vi "Editor Soglie.vi"(6 "delimiter":string="::", 7 "Grandezze misurate":string[](array[string]), 8 "file path Soglie int":path=path "C:/Lavori in corso/C2014015_CDR_PumpTEST/PC/Codice/Settings/Tolleranze misure/SoglieQH int.txt", 9 "file path Soglie costanti":path=path "C:/Lavori in corso/C2014015_CDR_PumpTEST/PC/Codice/Settings/Tolleranze misure/Soglie QH.txt", 10 "file path Soglie AQ int":path=path "C:/Lavori in corso/C2014015_CDR_PumpTEST/PC/Codice/Settings/Tolleranze misure/Soglie AQ QH int.txt", 11 "file path Soglie AQ costanti":path=path "C:/Lavori in corso/C2014015_CDR_PumpTEST/PC/Codice/Settings/Tolleranze misure/Soglie AQ QH.txt") -> (0 "Array soglie interpolate":T1(array[cluster]), 1 "Array soglie costanti":T2(array[cluster])=[{"Grandezza"="", "colonna"=1, "upper limit"=50.5, "misura"=0.0, "lower limit"=49.5, "Allarme?"=FALSE, "Inizio"=timestamp(0 s since 1904-01-01), "Durata [s]"=0.0}, {"Grandezza"="", "colonna"=2, "upper limit"=240.0, "misura"=0.0, "lower limit"=220.0, "Allarme?"=FALSE, "Inizio"=timestamp(0 s since 1904-01-01), "Durata [s]"=0.0}, {"Grandezza"="", "colonna"=3, "upper limit"=3.0, "misura"=0.0, "lower limit"=0.0, "Allarme?"=FALSE, "Inizio"=timestamp(0 s since 1904-01-01), "Durata [s]"=0.0}], 2 "Soglie AQ interpolate":T3(array[cluster]), 3 "Soglie AQ costanti":T4(array[cluster]))   [LabVIEW 2016]
uses:
  <vilib>/Utility/file.llb/Read From Spreadsheet File (string).vi
  <vilib>/Utility/file.llb/Write To Spreadsheet File (string).vi
  <vilib>/Utility/file.llb/Write To Spreadsheet File (DBL).vi
panel:
  in  "Intervento\nsoglie":bool caption="Soglia costante\n\nSoglia interpolata"
  out "Grandezza\nselezionata":string
  in  "Selezione\nsoglie":bool caption="Soglia costante\n\nSoglia interpolata"
  in  "Stop":bool
  in  "Soglia":T5 caption="Soglia costante"
  in  "Soglia interpolata":T6 caption="Soglia dinamica"
  in  "Grandezze misurate":i32(listbox)
  # "Soglie costanti"
  # "Soglie dinamiche"
  # "Solo acquisizione"
  # "Sempre attivo"
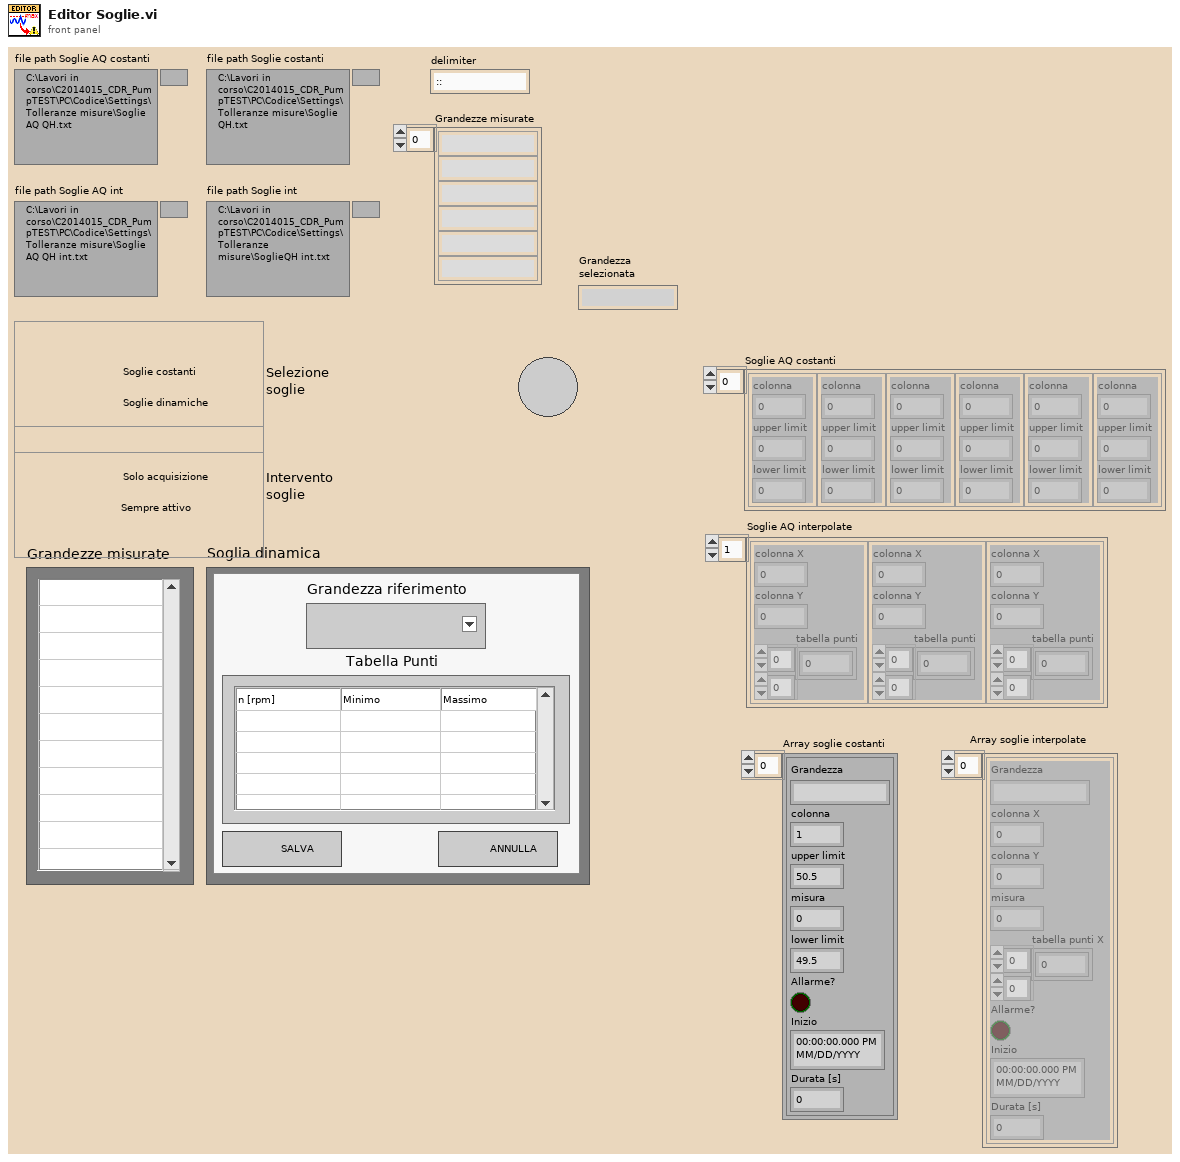
[diagram p1: front panel]
types:
  T1 = cluster{"Grandezza":string, "colonna X":i32, "colonna Y":i32, "misura":dbl, "tabella punti X":dbl[][], "Allarme?":bool, "Inizio":timestamp, "Durata [s]":dbl}[]
  T2 = cluster{"Grandezza":string, "colonna":i32, "upper limit":dbl, "misura":dbl, "lower limit":dbl, "Allarme?":bool, "Inizio":timestamp, "Durata [s]":dbl}[]
  T3 = cluster{"colonna X":i32, "colonna Y":i32, "tabella punti":dbl[][]}[]
  T4 = cluster{"colonna":i32, "upper limit":dbl, "lower limit":dbl}[]
  T5 = cluster{"Limite Massimo":dbl, "Limite Minimo":dbl, "Ok":bool, "ANNULLA":bool}
  T6 = cluster{"Tabella Punti":string[][], "Ok":bool, "ANNULLA":bool, "Grandezza riferimento":u16}
  T7 = cluster{"colonna X":i32, "colonna Y":i32, "tabella punti":dbl[][]}
  T8 = cluster{"colonna":i32, "upper limit":dbl, "lower limit":dbl}
  T9 = cluster{"Grandezza":string, "colonna X":i32, "colonna Y":i32, "misura":dbl, "tabella punti X":dbl[][], "Allarme?":bool, "Inizio":timestamp, "Durata [s]":dbl}
  T10 = cluster{"Grandezza":string, "colonna":i32, "upper limit":dbl, "misura":dbl, "lower limit":dbl, "Allarme?":bool, "Inizio":timestamp, "Durata [s]":dbl}
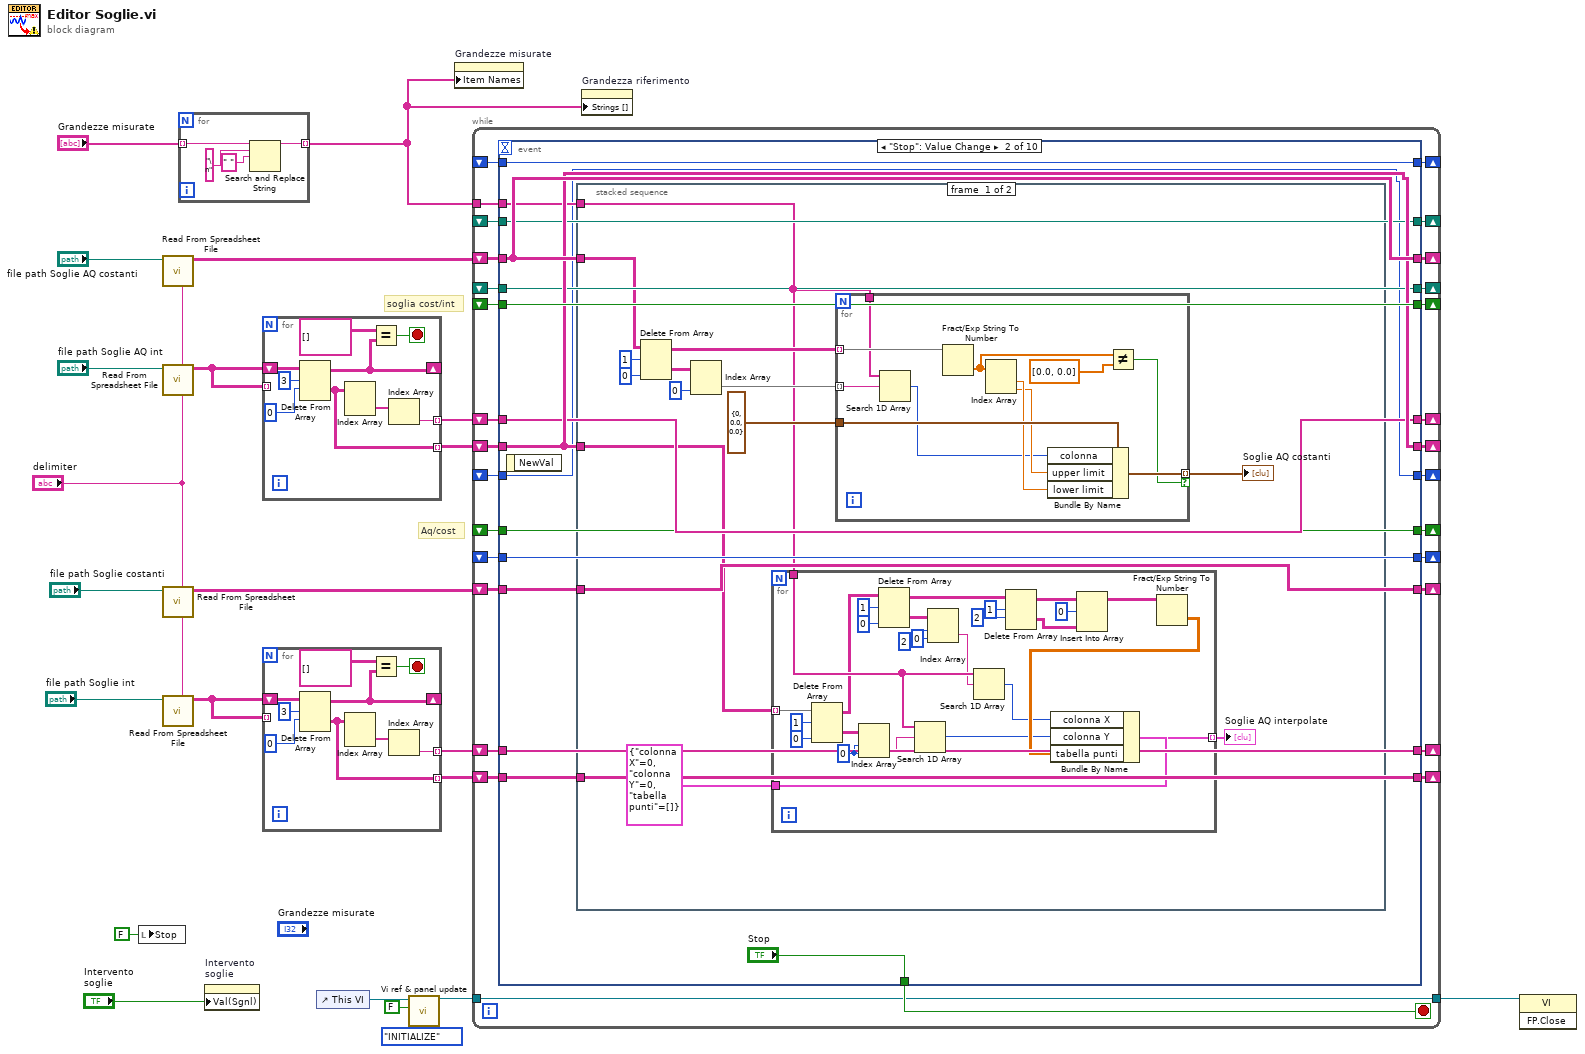
[diagram p0: block diagram]
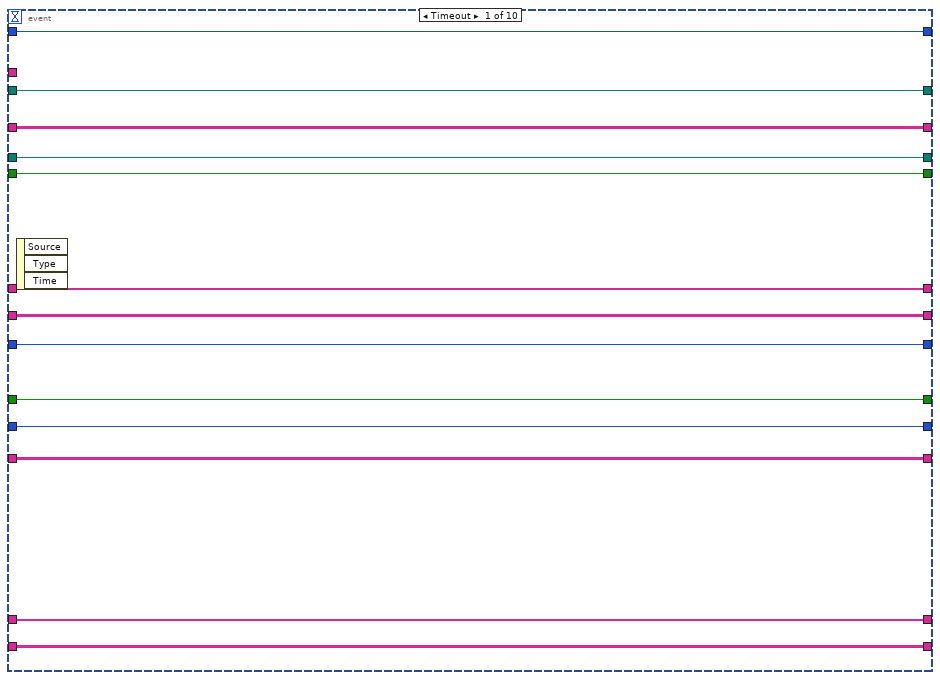
[diagram p2: hidden frame]
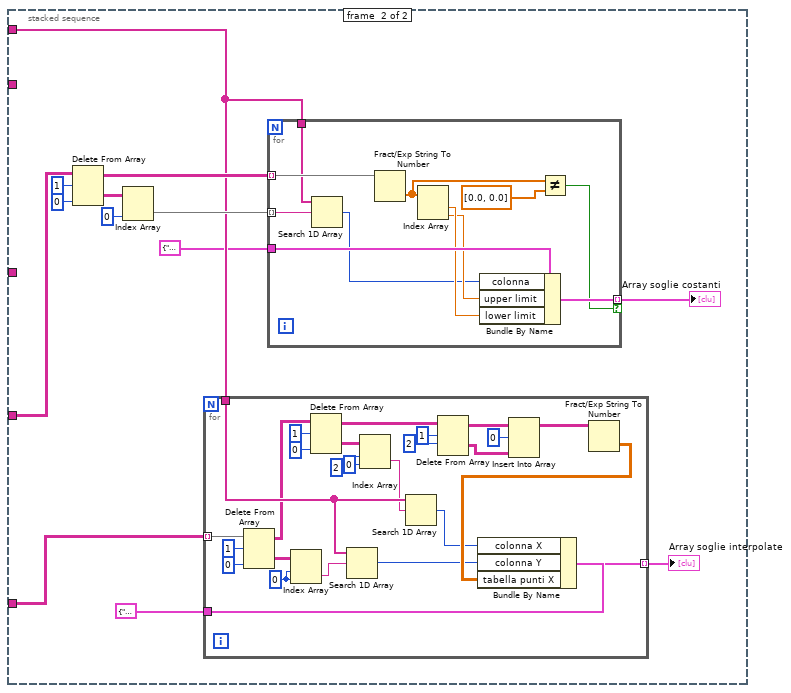
[diagram p3: hidden frame]
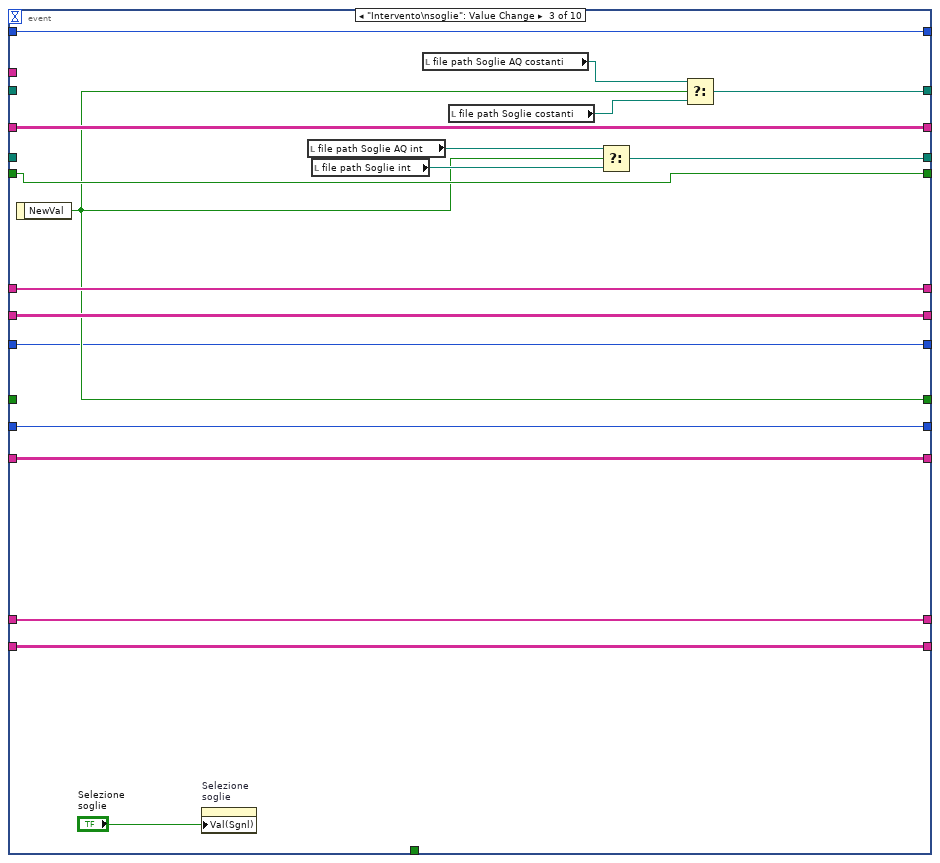
[diagram p4: hidden frame]
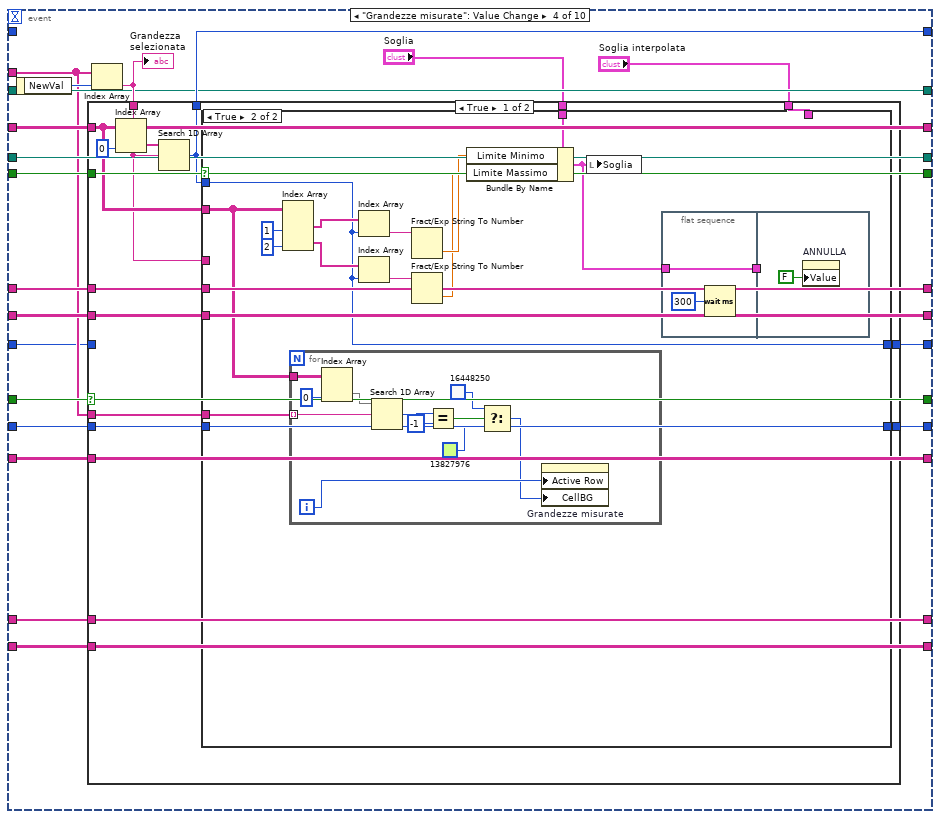
[diagram p5: hidden frame]
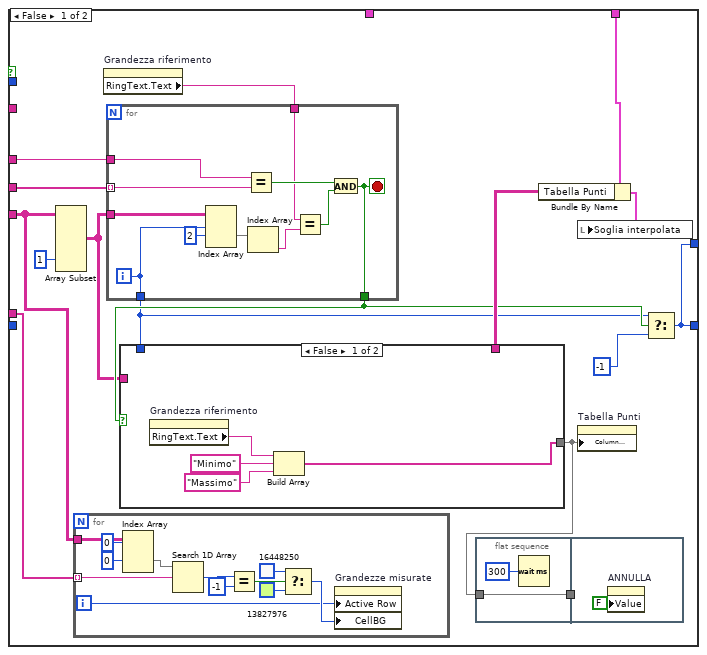
[diagram p6: hidden frame]
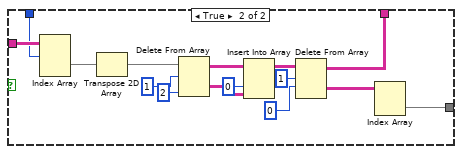
[diagram p7: hidden frame]
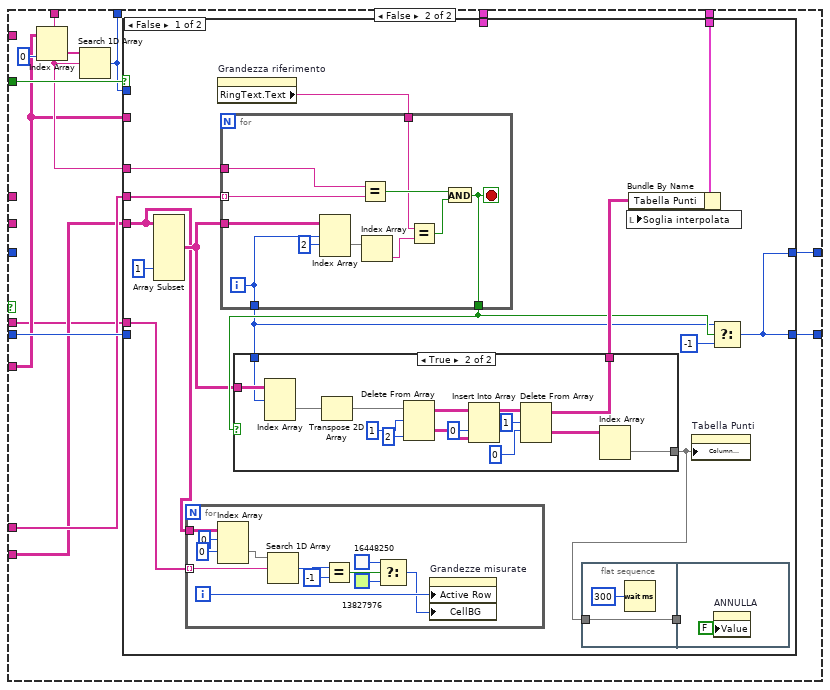
[diagram p8: hidden frame]
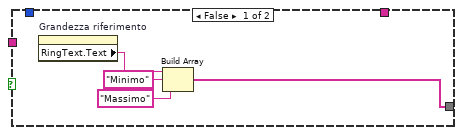
[diagram p9: hidden frame]
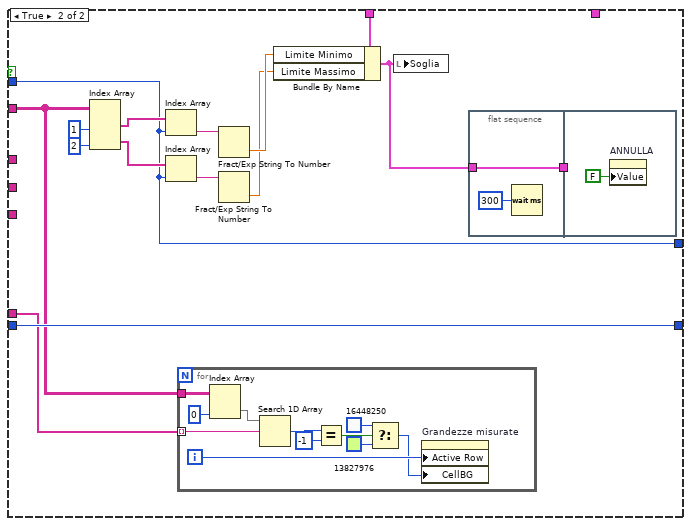
[diagram p10: hidden frame]
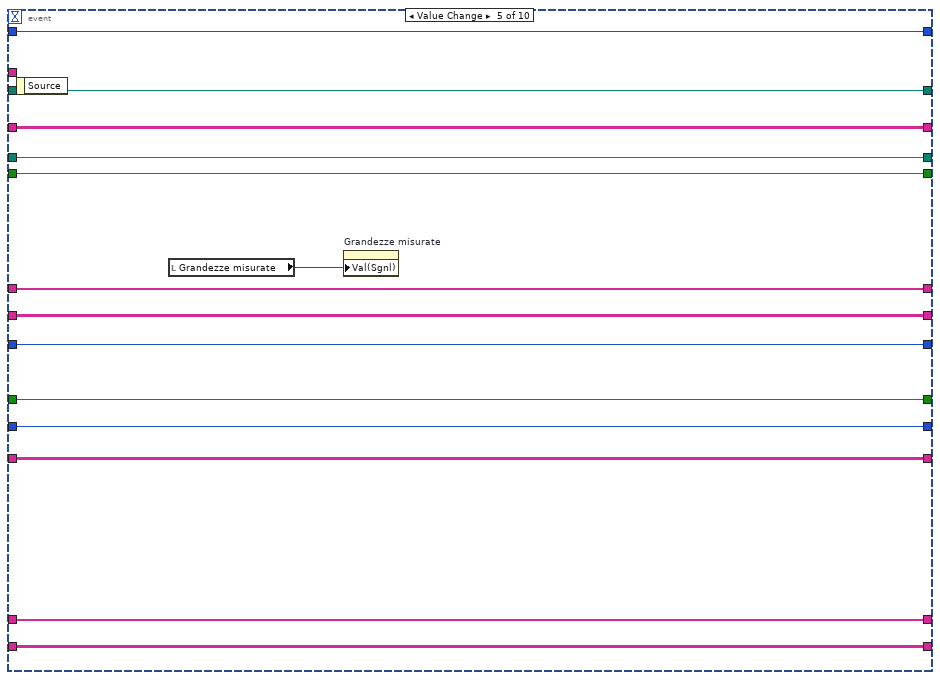
[diagram p11: hidden frame]
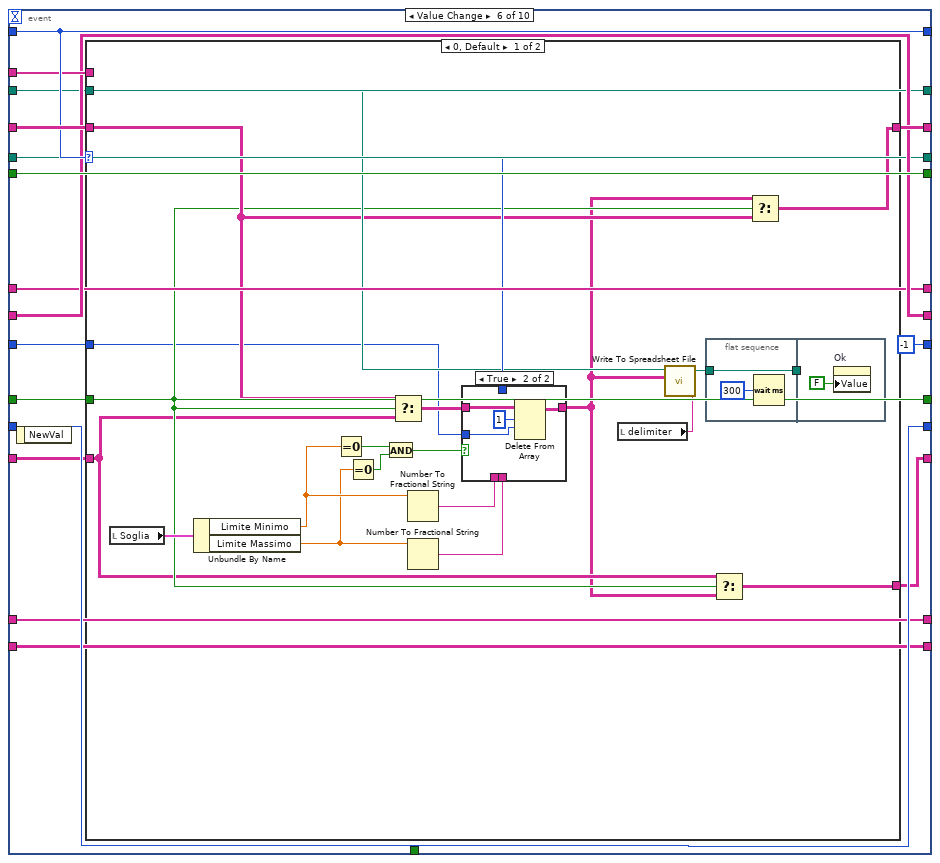
[diagram p12: hidden frame]
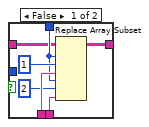
[diagram p13: hidden frame]
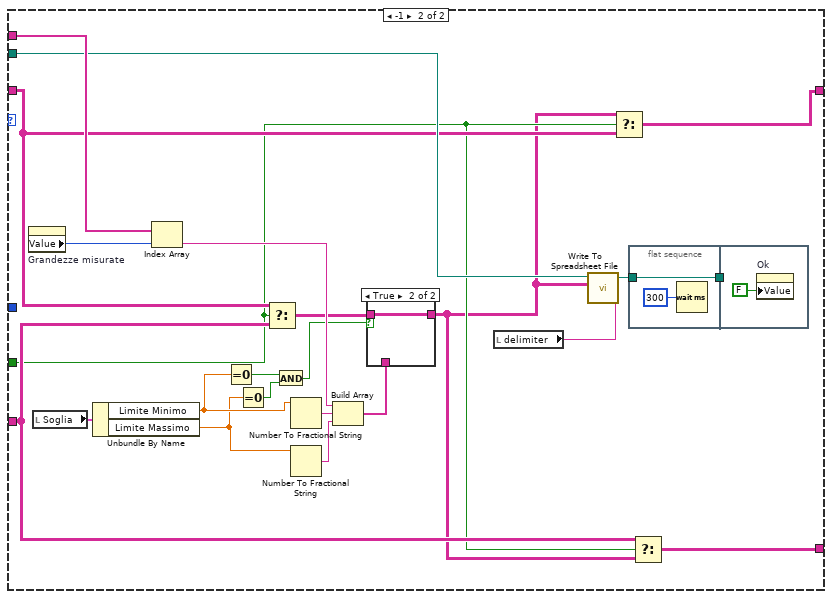
[diagram p14: hidden frame]
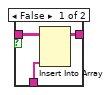
[diagram p15: hidden frame]
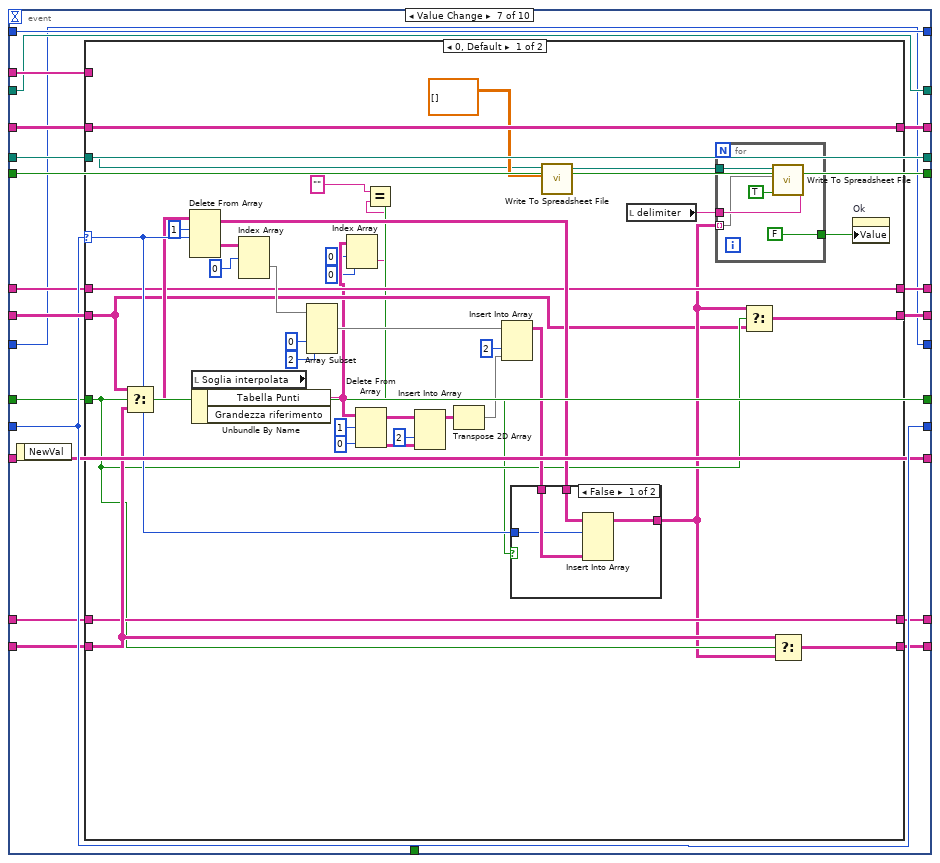
[diagram p16: hidden frame]
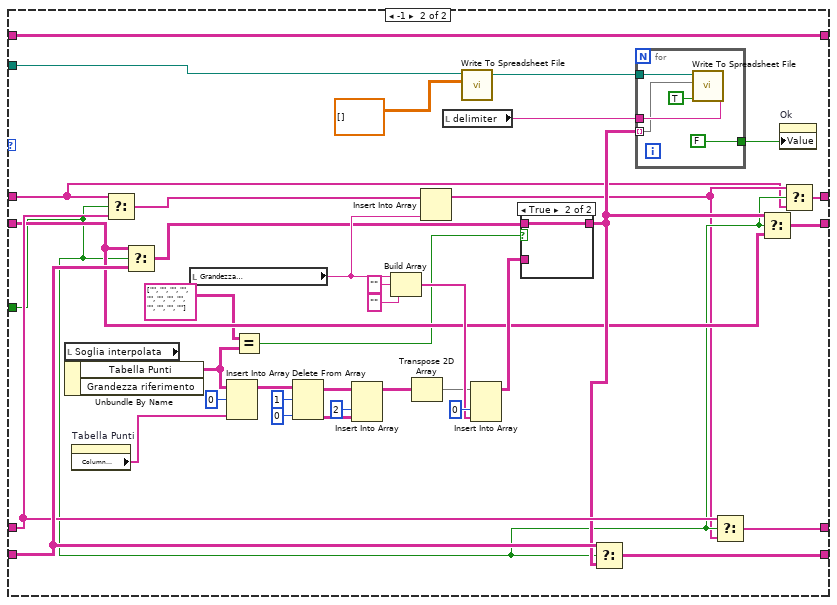
[diagram p18: hidden frame]
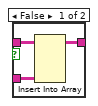
[diagram p19: hidden frame]
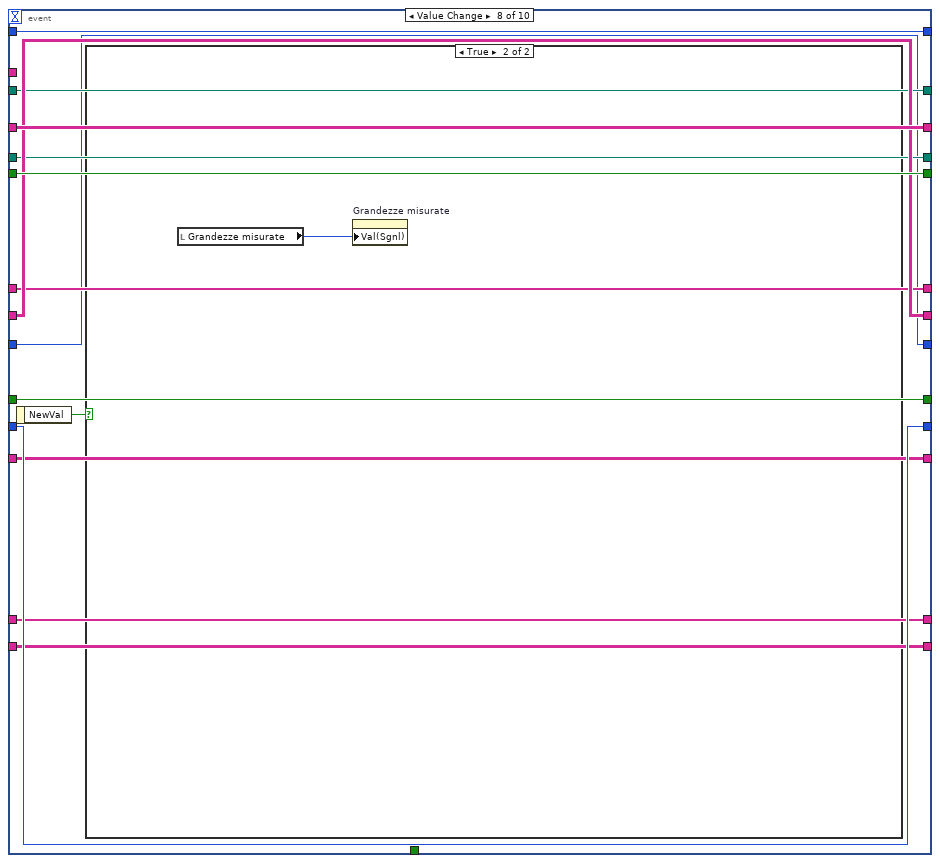
[diagram p20: hidden frame]
diagram:
  # "Aq/cost"
  # "soglia cost/int"
  n1 = local write "Stop"(FALSE ("Stop")) -> ()
  n2 = call-poly <vilib>:"Read From Spreadsheet File.vi"("delimiter (\\t)"="delimiter", "file path (dialog if empty)"="file path Soglie AQ costanti") -> ("all rows"=w12:string[][])  [unwired: 5 in, 4 out]
  n3 = call-poly <vilib>:"Read From Spreadsheet File.vi"("delimiter (\\t)"="delimiter", "file path (dialog if empty)"="file path Soglie AQ int") -> ("all rows"=w13:string[][])  [unwired: 5 in, 4 out]
  n4 = call-poly <vilib>:"Read From Spreadsheet File.vi"("delimiter (\\t)"="delimiter", "file path (dialog if empty)"="file path Soglie costanti") -> ("all rows"=w6:string[][])  [unwired: 5 in, 4 out]
  n5 = call-poly <vilib>:"Read From Spreadsheet File.vi"("delimiter (\\t)"="delimiter", "file path (dialog if empty)"="file path Soglie int") -> ("all rows"=w9:string[][])  [unwired: 5 in, 4 out]
  n6 = for {
    tunnel: "Grandezze misurate" -> [w26] mode=indexing
    tunnel: [w24] -> w1 mode=indexing
    n7 = Search and Replace String(input string=w26, search string="\n", replace string=" " ("replace string (\"\")")) -> (result string=w24:string)  [unwired: 5 in, 3 out]
  }
  n8 = property on="Intervento\nsoglie" class="Bool (strict)"("Val(Sgnl)"="Intervento\nsoglie") -> ()  [unwired: 2 in, 2 out]
  n9 = for {
    shift-right: [w31] -> _
    shift-left: w13 -> [w35]
    tunnel: [w29] -> w10 mode=indexing
    tunnel: [w27] -> w11 mode=indexing
    tunnel: w13 -> [_] mode=indexing
    stop <- w32 stop-if-true
    n10 = Delete From Array(array=w35, length=3, index (row)=0) -> (deleted portion=w27:string[][], array with subset deleted=w31:string[][])  [unwired: 1 in]
    n11 = Index Array(array=w27) -> (element=w30:string[])  [unwired: 2 in]
    n12 = Equal?(x=string[][] [] ("y"), y=w31) -> (x = y?=w32:bool)
    n13 = Index Array(array=w30) -> (element=w29:string)  [unwired: 1 in]
  }
  n14 = for {
    shift-right: [w40] -> _
    shift-left: w9 -> [w44]
    tunnel: [w38] -> w4 mode=indexing
    tunnel: [w36] -> w3 mode=indexing
    tunnel: w9 -> [_] mode=indexing
    stop <- w41 stop-if-true
    n15 = Delete From Array(array=w44, length=3, index (row)=0) -> (deleted portion=w36:string[][], array with subset deleted=w40:string[][])  [unwired: 1 in]
    n16 = Index Array(array=w36) -> (element=w39:string[])  [unwired: 2 in]
    n17 = Equal?(x=string[][] [] ("y"), y=w40) -> (x = y?=w41:bool)
    n18 = Index Array(array=w39) -> (element=w38:string)  [unwired: 1 in]
  }
  n19 = control-ref of="This VI"() -> (w20:refnum<vi>)
  n20 = call "Vi ref & panel update.vi"("Function"=enum16{"INITIALIZE", "DEF UPDATE"}."INITIALIZE", "Defer Panel Updates"=FALSE, "VI ref in"=w20) -> ("VI ref out"=w18:refnum<vi>)  [unwired: 7 in, 1 out]
  n21 = property on="Grandezze misurate" class="LstBox (strict)"("Item Names"=w1) -> ()  [unwired: 2 in, 2 out]
  n22 = while {
    shift-right: [w72] -> _
    shift-left: _ -> [w71]
    shift-right: [w69] -> _
    shift-left: w12 -> [w70]
    tunnel: w1 -> [w68]
    shift-right: [w67] -> _
    shift-left: _ -> [w66]
    shift-right: [w63] -> _
    shift-left: _ -> [w62]
    shift-right: [w61] -> _
    shift-left: w11 -> [w65]
    tunnel: w18 -> [w60]
    tunnel: [w60] -> w17
    shift-right: [w59] -> _
    shift-left: w10 -> [w64]
    shift-right: [w58] -> _
    shift-left: _ -> [w57]
    shift-right: [w56] -> _
    shift-left: _ -> [w55]
    shift-right: [w53] -> _
    shift-left: w4 -> [w52]
    shift-right: [w51] -> _
    shift-left: w3 -> [w50]
    shift-right: [w49] -> _
    shift-left: w6 -> [w54]
    shift-right: [w48] -> _
    shift-left: _ -> [w47]
    shift-right: [w46] -> _
    shift-left: _ -> [w45]
    stop <- w73 stop-if-true
    n23 = event shown="[1] \"Stop\": Value Change" {
      selector: _ -> [_ _ _ _ _ _ _ _ _ _]
      dyn-events: _ -> [_ _ _ _ _ _ _ _ _ _]
      timeout: _ -> [_ _ _ _ _ _ _ _ _ _]
      tunnel: [_ "Stop" _ _ _ _ _ _ _ _] -> w73
      tunnel: [w86 w100 w208 w239 w461 w478 w562 w674 w689 w705] -> w72
      tunnel: w71 -> [w86 w100 w208 w239 w461 w478 w562 w674 w689 _]
      tunnel: w70 -> [w85 w97 w217 w237 w460 w477 w561 w673 w688 w702]
      tunnel: [w85 w97 w217 w237 w460 w476 w560 w673 w688 w702] -> w69
      tunnel: w68 -> [_ w95 _ w222 _ w474 w558 _ _ _]
      tunnel: [w84 w99 w219 w236 w459 w475 w559 w671 w686 w701] -> w67
      tunnel: w66 -> [w84 w99 w219 _ w459 w475 w559 w671 w686 w701]
      tunnel: w65 -> [w82 w96 w215 w235 w456 w472 w557 w669 w684 w699]
      tunnel: w64 -> [w81 w94 w216 w231 w455 w471 w555 w668 w683 w698]
      tunnel: [w83 w98 w218 w233 w457 w473 w556 w670 w685 w700] -> w63
      tunnel: w62 -> [w83 w98 w218 w232 w457 w473 w556 w670 w685 w700]
      tunnel: [w82 w96 w215 w235 w456 w472 w545 w669 w684 w699] -> w61
      tunnel: [w81 w94 w216 w231 w455 w471 w547 w668 w683 w698] -> w59
      tunnel: [w80 w93 w212 w230 w454 w469 w554 w667 w682 w697] -> w58
      tunnel: w57 -> [w80 w93 _ w230 w454 w469 w554 w667 w682 w697]
      tunnel: [w79 w92 w209 w229 w453 w470 w553 w666 w681 w696] -> w56
      tunnel: w55 -> [w79 w92 _ w229 w453 w470 w553 w666 w681 w696]
      tunnel: w54 -> [w76 w89 w204 w225 w450 w465 w552 w663 w678 w693]
      tunnel: w52 -> [w78 w91 w206 w224 w452 w468 w550 w665 w680 w695]
      tunnel: w50 -> [w77 w88 w205 w223 w451 w467 w549 w664 w679 w694]
      tunnel: [w78 w91 w206 w224 w452 w468 w546 w665 w680 w695] -> w53
      tunnel: [w77 w88 w205 w223 w451 w467 w548 w664 w679 w694] -> w51
      tunnel: [w76 w89 w204 w225 w450 w464 w552 w663 w678 w693] -> w49
      tunnel: [w75 w90 w203 w226 w449 w466 w551 w662 w677 w692] -> w48
      tunnel: w47 -> [w75 w90 _ w226 w449 w466 w551 w662 w677 w692]
      tunnel: [w74 w87 w202 w221 w448 -1 ("index of element") w544 w661 w676 w691] -> w46
      tunnel: w45 -> [w74 w87 w202 w220 w448 w463 w544 w661 w676 w691]
      event Timeout {
        n24 = event-data() -> ()  [unwired: 1 in, 3 out]
      }
      event "Stop": Value Change {
        n25 = event-data() -> ()  [unwired: 1 in, 1 out]
        n26 = stacked-sequence {
          tunnel: w97 -> [w112 _]
          tunnel: w96 -> [w105 _]
          tunnel: w95 -> [w103 w158]
          tunnel: w89 -> [_ w157]
          tunnel: w88 -> [_ w156]
          frame #0 {
            n27 = Delete From Array(array=w112, length=1, index (col)=0 ("disabled index (col)")) -> (deleted portion=w108:string[][], array with subset deleted=w109:string[][])  [unwired: 1 in]
            n28 = Index Array(array=w108, index (col)=0 ("disabled index (col)")) -> (element=w107:string[])  [unwired: 1 in]
            n29 = for {
              tunnel: w105 -> [w139] mode=indexing
              tunnel: T7 {"colonna X"=0, "colonna Y"=0, "tabella punti"=[]} ("Soglie interpolate 2") -> [w140]
              tunnel: w103 -> [w129]
              tunnel: [w117] -> w102 mode=indexing
              w135 = 0 ("disabled index (col)")
              n30 = Delete From Array(array=w139, length=1, index (col)=0 ("disabled index (col)")) -> (deleted portion=w132:string[][], array with subset deleted=w126:string[][])  [unwired: 1 in]
              n31 = Index Array(array=w132, index (row)=w135, index (col)=w135) -> (element=w136:string)
              n32 = Delete From Array(array=w126, length=1, index (col)=0 ("disabled index (col)")) -> (deleted portion=w131:string[][], array with subset deleted=w125:string[][])  [unwired: 1 in]
              n33 = Search 1D Array(1D array=w129, element=w136) -> (index of element=w115:i32)  [unwired: 1 in]
              n34 = Index Array(array=w131, index (row)=2, index (col)=0 ("disabled index (col)")) -> (element=w127:string)
              n35 = Search 1D Array(1D array=w129, element=w127) -> (index of element=w116:i32)  [unwired: 1 in]
              n36 = Delete From Array(array=w125, length=1, index (row)=2) -> (deleted portion=w121:string[][], array with subset deleted=w122:string[][])  [unwired: 1 in]
              n37 = Insert Into Array(array=w122, index (row)=0, new element=w121) -> (w119:string[][])  [unwired: 1 in]
              n38 = Fract/Exp String To Number(string=w119) -> (number=w118:dbl[][])  [unwired: 3 in, 1 out]
              n39 = Bundle By Name(cluster=w140, "colonna X"=w116, "colonna Y"=w115, "tabella punti"=w118) -> (w117:T7)
            }
            "Soglie AQ interpolate" <- w102
            n40 = for {
              tunnel: T8 {"colonna"=0, "upper limit"=0.0, "lower limit"=0.0} ("Soglie costanti") -> [w151]
              tunnel: w109 -> [w150] mode=indexing
              tunnel: [w147] -> w113 mode=indexing if=w144
              tunnel: w103 -> [w143]
              tunnel: w107 -> [w142] mode=indexing
              n41 = Search 1D Array(1D array=w143, element=w142) -> (index of element=w141:i32)  [unwired: 1 in]
              n42 = Fract/Exp String To Number(string=w150) -> (number=w146:dbl[])  [unwired: 3 in, 1 out]
              n43 = Index Array(array=w146) -> (element #1=w149:dbl, element #2=w148:dbl)  [unwired: 2 in]
              n44 = Bundle By Name(cluster=w151, "colonna"=w141, "upper limit"=w148, "lower limit"=w149) -> (w147:T8)
              n45 = Not Equal?(x=w146, y=dbl[] [0.0, 0.0]) -> (x != y?=w144:bool)
            }
            "Soglie AQ costanti" <- w113
          }
          frame #1 {
            n46 = Delete From Array(array=w157, length=1, index (col)=0 ("disabled index (col)")) -> (deleted portion=w161:string[][], array with subset deleted=w162:string[][])  [unwired: 1 in]
            n47 = Index Array(array=w161, index (col)=0 ("disabled index (col)")) -> (element=w160:string[])  [unwired: 1 in]
            n48 = for {
              tunnel: w156 -> [w189] mode=indexing
              tunnel: T9 {"Grandezza"="", "colonna X"=0, "colonna Y"=0, "misura"=0.0, "tabella punti X"=[], "Allarme?"=FALSE, "Inizio"=timestamp(0 s since 1904-01-01), "Durata [s]"=0.0} ("soglie interpolate") -> [w190]
              tunnel: w158 -> [w179]
              tunnel: [w167] -> w152 mode=indexing
              w185 = 0 ("disabled index (col)")
              n49 = Delete From Array(array=w189, length=1, index (col)=0 ("disabled index (col)")) -> (deleted portion=w182:string[][], array with subset deleted=w176:string[][])  [unwired: 1 in]
              n50 = Index Array(array=w182, index (row)=w185, index (col)=w185) -> (element=w186:string)
              n51 = Delete From Array(array=w176, length=1, index (col)=0 ("disabled index (col)")) -> (deleted portion=w181:string[][], array with subset deleted=w175:string[][])  [unwired: 1 in]
              n52 = Search 1D Array(1D array=w179, element=w186) -> (index of element=w165:i32)  [unwired: 1 in]
              n53 = Index Array(array=w181, index (row)=2, index (col)=0 ("disabled index (col)")) -> (element=w177:string)
              n54 = Search 1D Array(1D array=w179, element=w177) -> (index of element=w166:i32)  [unwired: 1 in]
              n55 = Delete From Array(array=w175, length=1, index (row)=2) -> (deleted portion=w171:string[][], array with subset deleted=w172:string[][])  [unwired: 1 in]
              n56 = Insert Into Array(array=w172, index (row)=0, new element=w171) -> (w169:string[][])  [unwired: 1 in]
              n57 = Fract/Exp String To Number(string=w169) -> (number=w168:dbl[][])  [unwired: 3 in, 1 out]
              n58 = Bundle By Name(cluster=w190, "colonna X"=w166, "colonna Y"=w165, "tabella punti X"=w168) -> (w167:T9)
            }
            "Array soglie interpolate" <- w152
            n59 = for {
              tunnel: T10 {"Grandezza"="", "colonna"=1, "upper limit"=50.5, "misura"=0.0, "lower limit"=49.5, "Allarme?"=FALSE, "Inizio"=timestamp(0 s since 1904-01-01), "Durata [s]"=0.0} ("Cluster") -> [w201]
              tunnel: w162 -> [w200] mode=indexing
              tunnel: [w197] -> w154 mode=indexing if=w194
              tunnel: w158 -> [w193]
              tunnel: w160 -> [w192] mode=indexing
              n60 = Search 1D Array(1D array=w193, element=w192) -> (index of element=w191:i32)  [unwired: 1 in]
              n61 = Fract/Exp String To Number(string=w200) -> (number=w196:dbl[])  [unwired: 3 in, 1 out]
              n62 = Index Array(array=w196) -> (element #1=w199:dbl, element #2=w198:dbl)  [unwired: 2 in]
              n63 = Bundle By Name(cluster=w201, "colonna"=w191, "upper limit"=w198, "lower limit"=w199) -> (w197:T10)
              n64 = Not Equal?(x=w196, y=dbl[] [0.0, 0.0]) -> (x != y?=w194:bool)
            }
            "Array soglie costanti" <- w154
          }
        }
      }
      event "Intervento\nsoglie": Value Change {
        n65 = event-data() -> ("NewVal"=w203:bool)  [unwired: 1 in]
        n66 = property on="Selezione\nsoglie" class="Bool (strict)"("Val(Sgnl)"="Selezione\nsoglie") -> ()  [unwired: 2 in, 2 out]
        n67 = local read "file path Soglie AQ int"() -> (w210:path)
        n68 = local read "file path Soglie int"() -> (w211:path)
        n69 = local read "file path Soglie AQ costanti"() -> (w214:path)
        n70 = local read "file path Soglie costanti"() -> (w213:path)
        n71 = Select(t=w210, s=w203, f=w211) -> (s? t:f=w209:path)
        n72 = Select(t=w214, s=w203, f=w213) -> (s? t:f=w212:path)
      }
      event "Grandezze misurate": Value Change {
        n73 = event-data() -> ("NewVal"=w238:i32)  [unwired: 1 in]
        n74 = Index Array(array=w222, index=w238) -> (element=w234:string)
        "Grandezza\nselezionata" <- w234
        n75 = case shown="True" w226 {
          tunnel: w239 -> [w253 w357]
          tunnel: w237 -> [w250 _]
          tunnel: [w249 w354] -> w236
          tunnel: w235 -> [w248 _]
          tunnel: w234 -> [w247 w353]
          tunnel: [w246 w352] -> w233
          tunnel: w232 -> [w245 w351]
          tunnel: w231 -> [w244 _]
          tunnel: "Soglia" -> [w243 w350]
          tunnel: "Soglia interpolata" -> [w242 w349]
          tunnel: w225 -> [_ w346]
          tunnel: w224 -> [_ w348]
          tunnel: w223 -> [_ w347]
          tunnel: w222 -> [w241 w344]
          tunnel: [w240 w345] -> w221
          tunnel: w220 -> [_ _]
          frame True {
            n76 = Index Array(array=w250, index (col)=0 ("disabled index (col)")) -> (element=w251:string[])  [unwired: 1 in]
            n77 = Search 1D Array(1D array=w251, element=w247) -> (index of element=w249:i32)  [unwired: 1 in]
            n78 = case shown="True" w253 {
              tunnel: w250 -> [_ w317]
              tunnel: w249 -> [_ w315]
              tunnel: w248 -> [w254 _]
              tunnel: w244 -> [w269 _]
              tunnel: w247 -> [w268 _]
              tunnel: [w258 w319] -> w246
              tunnel: w245 -> [_ w319]
              tunnel: w243 -> [_ w318]
              tunnel: w242 -> [w259 _]
              tunnel: w241 -> [w257 w316]
              tunnel: [w258 w315] -> w240
              frame False {
                n79 = Array Subset(array=w254, index (dim 2)=1 ("index")) -> (w256:string[][][])  [unwired: 5 in]
                n80 = for {
                  tunnel: w254 -> [w281]
                  tunnel: w257 -> [w279] mode=indexing
                  i -> [w272]
                  n81 = Index Array(array=w281, index (dim 1)=0 ("disabled index (row)"), index (dim 2)=0 ("disabled index (col)")) -> (element=w280:string[])  [unwired: 1 in]
                  n82 = Search 1D Array(1D array=w280, element=w279) -> (index of element=w278:i32)  [unwired: 1 in]
                  n83 = Equal?(x=w278, y=-1) -> (x = y?=w276:bool)
                  n84 = Select(t=u32 16448250, s=w276, f=u32 13827976) -> (s? t:f=w273:u32)
                  n85 = property on="Grandezze misurate" class="LstBox (strict)"("Active Row"=w272, "CellBG"=w273) -> ()  [unwired: 2 in, 2 out]
                }
                n86 = property on="Grandezza riferimento" class="Ring (strict)"() -> ("RingText.Text"=w267:string)  [unwired: 2 in, 2 out]
                n87 = for {
                  tunnel: w269 -> [w314] mode=indexing
                  tunnel: w268 -> [w313]
                  tunnel: w256 -> [w306]
                  tunnel: w267 -> [w308]
                  tunnel: [w305] -> w263
                  tunnel: [w304] -> w264
                  i -> [w305]
                  stop <- w304 stop-if-true
                  n88 = Index Array(array=w306, index (dim 0)=w305, index (dim 1)=2 ("disabled index (row)")) -> (element=w310:string[])  [unwired: 1 in]
                  n89 = Equal?(x=w313, y=w314) -> (x = y?=w312:bool)
                  n90 = Index Array(array=w310) -> (element=w309:string)  [unwired: 1 in]
                  n91 = Equal?(x=w308, y=w309) -> (x = y?=w307:bool)
                  n92 = And(x=w312, y=w307) -> (x .and. y?=w304:bool)
                }
                n93 = case shown="False" w264 {
                  tunnel: w256 -> [_ w303]
                  tunnel: w263 -> [_ w302]
                  tunnel: [w285 w292] -> w260
                  tunnel: [_ w291] -> w266
                  frame False {
                    n94 = property on="Grandezza riferimento" class="Ring (strict)"() -> ("RingText.Text"=w288:string)  [unwired: 2 in, 2 out]
                    n95 = Build Array(w288, "Minimo" ("element"), "Massimo" ("element")) -> (w285:string[])
                  }
                  frame True {
                    n96 = Index Array(array=w303, index (dim 0)=w302) -> (element=w290:string[][])  [unwired: 2 in]
                    n97 = Transpose 2D Array(2D array=w290) -> (transposed array=w289:string[][])
                    n98 = Delete From Array(array=w289, length=1, index (col)=2 ("disabled index (col)")) -> (deleted portion=w298:string[][], array with subset deleted=w299:string[][])  [unwired: 1 in]
                    n99 = Insert Into Array(array=w299, index (col)=0 ("disabled index (col)"), new element=w298) -> (w296:string[][])  [unwired: 1 in]
                    n100 = Delete From Array(array=w296, length=1, index (row)=0) -> (deleted portion=w293:string[][], array with subset deleted=w291:string[][])  [unwired: 1 in]
                    n101 = Index Array(array=w293) -> (element=w292:string[])  [unwired: 2 in]
                  }
                }
                n102 = flat-sequence {
                  tunnel: w260 -> [w283]
                  tunnel: [w283] -> w261
                  tunnel: w261 -> [_]
                  frame #0 {
                    n103 = Wait (ms)(milliseconds to wait=u32 300) -> ()  [unwired: 1 out]
                  }
                  frame #1 {
                    n104 = property on="ANNULLA" class="Bool (strict)"("Value"=FALSE) -> ()  [unwired: 2 in, 2 out]
                  }
                }
                n105 = Bundle By Name(cluster=w259, "Tabella Punti"=w266) -> (w265:T6)
                n106 = local write "Soglia interpolata"(w265) -> ()
                n107 = property on="Tabella Punti" class="Tbl (strict)"("Column Headers[]"=w260) -> ()  [unwired: 2 in, 2 out]
                n108 = Select(t=w263, s=w264, f=-1) -> (s? t:f=w258:i32)
              }
              frame True {
                n109 = Index Array(array=w317, index (col) #1=1 ("disabled index (col)"), index (col) #2=2 ("index (col)")) -> (element #1=w327:string[], element #2=w326:string[])  [unwired: 2 in]
                n110 = for {
                  tunnel: w317 -> [w340]
                  tunnel: w316 -> [w337] mode=indexing
                  i -> [w336]
                  n111 = Index Array(array=w340, index (col)=0 ("disabled index (col)")) -> (element=w338:string[])  [unwired: 1 in]
                  n112 = Search 1D Array(1D array=w338, element=w337) -> (index of element=w335:i32)  [unwired: 1 in]
                  n113 = Equal?(x=w335, y=-1) -> (x = y?=w333:bool)
                  n114 = Select(t=u32 16448250, s=w333, f=u32 13827976) -> (s? t:f=w330:u32)
                  n115 = property on="Grandezze misurate" class="LstBox (strict)"("Active Row"=w336, "CellBG"=w330) -> ()  [unwired: 2 in, 2 out]
                }
                n116 = Index Array(array=w327, index=w315) -> (element=w325:string)
                n117 = Index Array(array=w326, index=w315) -> (element=w323:string)
                n118 = Fract/Exp String To Number(string=w325) -> (number=w324:dbl)  [unwired: 3 in, 1 out]
                n119 = Fract/Exp String To Number(string=w323) -> (number=w322:dbl)  [unwired: 3 in, 1 out]
                n120 = Bundle By Name(cluster=w318, "Limite Minimo"=w324, "Limite Massimo"=w322) -> (w321:T5)
                n121 = local write "Soglia"(w321) -> ()
                n122 = flat-sequence {
                  tunnel: w321 -> [w342]
                  tunnel: [w342] -> w320
                  tunnel: w320 -> [_]
                  frame #0 {
                    n123 = Wait (ms)(milliseconds to wait=u32 300) -> ()  [unwired: 1 out]
                  }
                  frame #1 {
                    n124 = property on="ANNULLA" class="Bool (strict)"("Value"=FALSE) -> ()  [unwired: 2 in, 2 out]
                  }
                }
              }
            }
          }
          frame False {
            n125 = Index Array(array=w346, index (col)=0 ("disabled index (col)")) -> (element=w355:string[])  [unwired: 1 in]
            n126 = Search 1D Array(1D array=w355, element=w353) -> (index of element=w354:i32)  [unwired: 1 in]
            n127 = case shown="False" w357 {
              tunnel: w346 -> [_ w420]
              tunnel: w354 -> [_ w421]
              tunnel: w347 -> [w358 _]
              tunnel: w348 -> [w373 _]
              tunnel: w353 -> [w372 _]
              tunnel: [w361 w423] -> w352
              tunnel: w351 -> [_ w423]
              tunnel: w350 -> [_ w422]
              tunnel: w349 -> [w362 _]
              tunnel: [w361 w421] -> w345
              tunnel: w344 -> [w359 w419]
              frame False {
                n128 = Array Subset(array=w358, index (dim 2)=1 ("index")) -> (w360:string[][][])  [unwired: 5 in]
                n129 = for {
                  tunnel: w358 -> [w385]
                  tunnel: w359 -> [w382] mode=indexing
                  i -> [w381]
                  n130 = Index Array(array=w385, index (dim 1)=0 ("disabled index (col)"), index (dim 2)=0 ("disabled index (col)")) -> (element=w383:string[])  [unwired: 1 in]
                  n131 = Search 1D Array(1D array=w383, element=w382) -> (index of element=w380:i32)  [unwired: 1 in]
                  n132 = Equal?(x=w380, y=-1) -> (x = y?=w378:bool)
                  n133 = Select(t=u32 16448250, s=w378, f=u32 13827976) -> (s? t:f=w375:u32)
                  n134 = property on="Grandezze misurate" class="LstBox (strict)"("Active Row"=w381, "CellBG"=w375) -> ()  [unwired: 2 in, 2 out]
                }
                n135 = property on="Grandezza riferimento" class="Ring (strict)"() -> ("RingText.Text"=w371:string)  [unwired: 2 in, 2 out]
                n136 = for {
                  tunnel: w373 -> [w418] mode=indexing
                  tunnel: w372 -> [w417]
                  tunnel: w360 -> [w410]
                  tunnel: w371 -> [w412]
                  tunnel: [w409] -> w366
                  tunnel: [w408] -> w367
                  i -> [w409]
                  stop <- w408 stop-if-true
                  n137 = Index Array(array=w410, index (dim 0)=w409, index (dim 1)=2 ("disabled index (row)")) -> (element=w414:string[])  [unwired: 1 in]
                  n138 = Equal?(x=w417, y=w418) -> (x = y?=w416:bool)
                  n139 = Index Array(array=w414) -> (element=w413:string)  [unwired: 1 in]
                  n140 = Equal?(x=w412, y=w413) -> (x = y?=w411:bool)
                  n141 = And(x=w416, y=w411) -> (x .and. y?=w408:bool)
                }
                n142 = case shown="True" w367 {
                  tunnel: w360 -> [_ w407]
                  tunnel: w366 -> [_ w406]
                  tunnel: [w389 w396] -> w363
                  tunnel: [_ w395] -> w370
                  frame False {
                    n143 = property on="Grandezza riferimento" class="Ring (strict)"() -> ("RingText.Text"=w392:string)  [unwired: 2 in, 2 out]
                    n144 = Build Array(w392, "Minimo" ("element"), "Massimo" ("element")) -> (w389:string[])
                  }
                  frame True {
                    n145 = Index Array(array=w407, index (dim 0)=w406) -> (element=w394:string[][])  [unwired: 2 in]
                    n146 = Transpose 2D Array(2D array=w394) -> (transposed array=w393:string[][])
                    n147 = Delete From Array(array=w393, length=1, index (col)=2 ("disabled index (col)")) -> (deleted portion=w402:string[][], array with subset deleted=w403:string[][])  [unwired: 1 in]
                    n148 = Insert Into Array(array=w403, index (col)=0 ("disabled index (col)"), new element=w402) -> (w400:string[][])  [unwired: 1 in]
                    n149 = Delete From Array(array=w400, length=1, index (row)=0) -> (deleted portion=w397:string[][], array with subset deleted=w395:string[][])  [unwired: 1 in]
                    n150 = Index Array(array=w397) -> (element=w396:string[])  [unwired: 2 in]
                  }
                }
                n151 = flat-sequence {
                  tunnel: w363 -> [w387]
                  tunnel: [w387] -> w364
                  tunnel: w364 -> [_]
                  frame #0 {
                    n152 = Wait (ms)(milliseconds to wait=u32 300) -> ()  [unwired: 1 out]
                  }
                  frame #1 {
                    n153 = property on="ANNULLA" class="Bool (strict)"("Value"=FALSE) -> ()  [unwired: 2 in, 2 out]
                  }
                }
                n154 = Bundle By Name(cluster=w362, "Tabella Punti"=w370) -> (w369:T6)
                n155 = local write "Soglia interpolata"(w369) -> ()
                n156 = property on="Tabella Punti" class="Tbl (strict)"("Column Headers[]"=w363) -> ()  [unwired: 2 in, 2 out]
                n157 = Select(t=w366, s=w367, f=-1) -> (s? t:f=w361:i32)
              }
              frame True {
                n158 = Index Array(array=w420, index (col) #1=1 ("disabled index (col)"), index (col) #2=2 ("index (col)")) -> (element #1=w431:string[], element #2=w430:string[])  [unwired: 2 in]
                n159 = Index Array(array=w431, index=w421) -> (element=w429:string)
                n160 = Index Array(array=w430, index=w421) -> (element=w427:string)
                n161 = for {
                  tunnel: w420 -> [w444]
                  tunnel: w419 -> [w441] mode=indexing
                  i -> [w440]
                  n162 = Index Array(array=w444, index (col)=0 ("disabled index (col)")) -> (element=w442:string[])  [unwired: 1 in]
                  n163 = Search 1D Array(1D array=w442, element=w441) -> (index of element=w439:i32)  [unwired: 1 in]
                  n164 = Equal?(x=w439, y=-1) -> (x = y?=w437:bool)
                  n165 = Select(t=u32 16448250, s=w437, f=u32 13827976) -> (s? t:f=w434:u32)
                  n166 = property on="Grandezze misurate" class="LstBox (strict)"("Active Row"=w440, "CellBG"=w434) -> ()  [unwired: 2 in, 2 out]
                }
                n167 = Fract/Exp String To Number(string=w429) -> (number=w428:dbl)  [unwired: 3 in, 1 out]
                n168 = Fract/Exp String To Number(string=w427) -> (number=w426:dbl)  [unwired: 3 in, 1 out]
                n169 = Bundle By Name(cluster=w422, "Limite Minimo"=w428, "Limite Massimo"=w426) -> (w425:T5)
                n170 = local write "Soglia"(w425) -> ()
                n171 = flat-sequence {
                  tunnel: w425 -> [w446]
                  tunnel: [w446] -> w424
                  tunnel: w424 -> [_]
                  frame #0 {
                    n172 = Wait (ms)(milliseconds to wait=u32 300) -> ()  [unwired: 1 out]
                  }
                  frame #1 {
                    n173 = property on="ANNULLA" class="Bool (strict)"("Value"=FALSE) -> ()  [unwired: 2 in, 2 out]
                  }
                }
              }
            }
          }
        }
      }
      event "Soglia interpolata.Grandezza riferimento": Value Change {
        n174 = event-data() -> ()  [unwired: 1 in, 1 out]
        n175 = local read "Grandezze misurate"() -> (w458:i32)
        n176 = property on="Grandezze misurate" class="LstBox (strict)"("Val(Sgnl)"=w458) -> ()  [unwired: 2 in, 2 out]
      }
      event "Soglia.Ok": Value Change {
        n177 = event-data() -> ()  [unwired: 1 in, 1 out]
        n178 = case shown="0, Default" w475 {
          selector: w475 -> [w493 _]
          tunnel: w477 -> [w489 w524]
          tunnel: [w490 w523] -> w476
          tunnel: w474 -> [_ w529]
          tunnel: w469 -> [w492 w526]
          tunnel: w466 -> [w488 w520]
          tunnel: w465 -> [w487 w522]
          tunnel: [w485 w521] -> w464
          tunnel: w463 -> [w479 _]
          frame 0, Default {
            n179 = local read "Soglia"() -> (w499:T5)
            n180 = Unbundle By Name(w499) -> ("Limite Minimo"=w482:dbl, "Limite Massimo"=w481:dbl)
            n181 = Equal To 0?(x=w482) -> (x = 0?=w483:bool)
            n182 = Equal To 0?(x=w481) -> (x = 0?=w484:bool)
            n183 = And(x=w483, y=w484) -> (x .and. y?=w480:bool)
            n184 = Select(t=w489, s=w488, f=w487) -> (s? t:f=w491:string[][])
            n185 = Number To Fractional String(number=w482) -> (F-format string=w498:string)  [unwired: 3 in]
            n186 = Number To Fractional String(number=w481) -> (F-format string=w497:string)  [unwired: 3 in]
            n187 = case shown="True" w480 {
              tunnel: w498 -> [w505 _]
              tunnel: w497 -> [w503 _]
              tunnel: w493 -> [w502 _]
              tunnel: w491 -> [w501 w510]
              tunnel: [w500 w509] -> w486
              tunnel: w479 -> [_ w507]
              frame False {
                n188 = Replace Array Subset(array=w501, new element #1=w505, index (row) #1=w502, index (col) #1=1 ("disabled index (col)"), new element #2=w503, index (row) #2=w502, index (col) #2=2 ("index (col)")) -> (w500:string[][])
              }
              frame True {
                n189 = Delete From Array(array=w510, length=1, index (row)=w507) -> (array with subset deleted=w509:string[][])  [unwired: 1 in, 1 out]
              }
            }
            n190 = local read "delimiter"() -> (w495:string)
            n191 = call-poly <vilib>:"Write To Spreadsheet File.vi"("delimiter (\\t)"=w495, "2D data"=w486, "file path (dialog if empty)"=w492) -> ("new file path (Not A Path if cancelled)"=w496:path)  [unwired: 5 in]
            n192 = flat-sequence {
              tunnel: w496 -> [w512]
              tunnel: [w512] -> w494
              tunnel: w494 -> [_]
              frame #0 {
                n193 = Wait (ms)(milliseconds to wait=u32 300) -> ()  [unwired: 1 out]
              }
              frame #1 {
                n194 = property on="Ok" class="Bool (strict)"("Value"=FALSE) -> ()  [unwired: 2 in, 2 out]
              }
            }
            n195 = Select(t=w487, s=w488, f=w486) -> (s? t:f=w485:string[][])
            n196 = Select(t=w486, s=w488, f=w489) -> (s? t:f=w490:string[][])
          }
          frame -1 {
            n197 = property on="Grandezze misurate" class="LstBox (strict)"() -> ("Value"=w528:i32)  [unwired: 2 in, 2 out]
            n198 = local read "Soglia"() -> (w536:T5)
            n199 = Unbundle By Name(w536) -> ("Limite Minimo"=w516:dbl, "Limite Massimo"=w515:dbl)
            n200 = Index Array(array=w529, index=w528) -> (element=w527:string)
            n201 = Equal To 0?(x=w516) -> (x = 0?=w517:bool)
            n202 = Equal To 0?(x=w515) -> (x = 0?=w518:bool)
            n203 = Select(t=w524, s=w520, f=w522) -> (s? t:f=w525:string[][])
            n204 = And(x=w517, y=w518) -> (x .and. y?=w514:bool)
            n205 = Number To Fractional String(number=w516) -> (F-format string=w532:string)  [unwired: 3 in]
            n206 = Number To Fractional String(number=w515) -> (F-format string=w530:string)  [unwired: 3 in]
            n207 = Build Array(w527, w532, w530) -> (w531:string[])
            n208 = case shown="True" w514 {
              tunnel: w531 -> [w539 _]
              tunnel: w525 -> [w538 w540]
              tunnel: [w537 w540] -> w519
              frame False {
                n209 = Insert Into Array(array=w538, new element=w539) -> (w537:string[][])  [unwired: 2 in]
              }
              frame True {
              }
            }
            n210 = local read "delimiter"() -> (w534:string)
            n211 = call-poly <vilib>:"Write To Spreadsheet File.vi"("delimiter (\\t)"=w534, "2D data"=w519, "file path (dialog if empty)"=w526) -> ("new file path (Not A Path if cancelled)"=w535:path)  [unwired: 5 in]
            n212 = Select(t=w519, s=w520, f=w524) -> (s? t:f=w523:string[][])
            n213 = flat-sequence {
              tunnel: w535 -> [w542]
              tunnel: [w542] -> w533
              tunnel: w533 -> [_]
              frame #0 {
                n214 = Wait (ms)(milliseconds to wait=u32 300) -> ()  [unwired: 1 out]
              }
              frame #1 {
                n215 = property on="Ok" class="Bool (strict)"("Value"=FALSE) -> ()  [unwired: 2 in, 2 out]
              }
            }
            n216 = Select(t=w522, s=w520, f=w519) -> (s? t:f=w521:string[][])
          }
        }
      }
      event "Soglia interpolata.Ok": Value Change {
        n217 = event-data() -> ()  [unwired: 1 in, 1 out]
        n218 = case shown="0, Default" w556 {
          selector: w556 -> [w583 _]
          tunnel: w561 -> [w586 w645]
          tunnel: [w586 w645] -> w560
          tunnel: w558 -> [_ _]
          tunnel: w557 -> [w569 w621]
          tunnel: [w570 w620] -> w545
          tunnel: w555 -> [w574 w617]
          tunnel: [w574 w616] -> w547
          tunnel: w553 -> [w578 w629]
          tunnel: w551 -> [w572 w619]
          tunnel: w550 -> [w573 w624]
          tunnel: w549 -> [w575 w626]
          tunnel: [w576 w625] -> w548
          tunnel: [w573 w623] -> w546
          frame 0, Default {
            n219 = Select(t=w569, s=w572, f=w575) -> (s? t:f=w577:string[][][])
            n220 = Delete From Array(array=w577, length=1, index (dim 0)=w583) -> (deleted portion=w594:string[][][], array with subset deleted=w584:string[][][])  [unwired: 2 in]
            n221 = local read "Soglia interpolata"() -> (w602:T6)
            n222 = Unbundle By Name(w602) -> ("Tabella Punti"=w567:string[][])  [unwired: 1 out]
            n223 = Index Array(array=w594, index (dim 0)=0 ("index (page)")) -> (element=w592:string[][])  [unwired: 2 in]
            n224 = Array Subset(array=w592, index (col)=0 ("index"), length (col)=2 ("length")) -> (w589:string[][])  [unwired: 2 in]
            n225 = Index Array(array=w567, index (row)=0, index (col)=0 ("disabled index (col)")) -> (element=w564:string)
            n226 = Delete From Array(array=w567, length=1, index (col)=0 ("disabled index (col)")) -> (deleted portion=w598:string[][], array with subset deleted=w599:string[][])  [unwired: 1 in]
            n227 = Equal?(x="", y=w564) -> (x = y?=w568:bool)
            n228 = Insert Into Array(array=w599, index (col)=2 ("disabled index (col)"), new element=w598) -> (w596:string[][])  [unwired: 1 in]
            n229 = Transpose 2D Array(2D array=w596) -> (transposed array=w588:string[][])
            n230 = Insert Into Array(array=w589, index (col)=2 ("disabled index (col)"), new element=w588) -> (w585:string[][])  [unwired: 1 in]
            n231 = case shown="False" w568 {
              tunnel: w585 -> [w606 _]
              tunnel: w584 -> [w605 w607]
              tunnel: w583 -> [w604 _]
              tunnel: [w603 w607] -> w571
              frame False {
                n232 = Insert Into Array(array=w605, index (dim 0)=w604, new element=w606) -> (w603:string[][][])  [unwired: 2 in]
              }
              frame True {
              }
            }
            n233 = call-poly <vilib>:"Write To Spreadsheet File.vi"("2D data"=dbl[][] [], "file path (dialog if empty)"=w578) -> ("new file path (Not A Path if cancelled)"=w579:path)  [unwired: 6 in]
            n234 = local read "delimiter"() -> (w581:string)
            n235 = for {
              tunnel: w579 -> [w612]
              tunnel: w581 -> [w611]
              tunnel: w571 -> [w610] mode=indexing
              tunnel: [FALSE ("append to file? (new file:F)")] -> w582
              n236 = call-poly <vilib>:"Write To Spreadsheet File.vi"("delimiter (\\t)"=w611, "append to file? (new file:F)"=TRUE, "2D data"=w610, "file path (dialog if empty)"=w612) -> ()  [unwired: 4 in, 1 out]
            }
            n237 = Select(t=w571, s=w572, f=w569) -> (s? t:f=w570:string[][][])
            n238 = Select(t=w575, s=w572, f=w571) -> (s? t:f=w576:string[][][])
            n239 = property on="Ok" class="Bool (strict)"("Value"=w582) -> ()  [unwired: 2 in, 2 out]
          }
          frame -1 {
            n240 = local read "Soglia interpolata"() -> (w651:T6)
            n241 = Unbundle By Name(w651) -> ("Tabella Punti"=w615:string[][])  [unwired: 1 out]
            n242 = property on="Tabella Punti" class="Tbl (strict)"() -> ("Column Headers[]"=w636:string[])  [unwired: 2 in, 2 out]
            n243 = Select(t=w617, s=w619, f=w624) -> (s? t:f=w628:string[])
            n244 = Select(t=w621, s=w619, f=w626) -> (s? t:f=w627:string[][][])
            n245 = local read "Grandezza\nselezionata"() -> (w630:string)
            n246 = Insert Into Array(array=w615, index (row)=0, new element=w636) -> (w637:string[][])  [unwired: 1 in]
            n247 = Equal?(x=string[][] [["", "", ""], ["", "", ""], ["", "", ""], ["", "", ""]] ("Tabella Punti"), y=w615) -> (x = y?=w613:bool)
            n248 = Delete From Array(array=w637, length=1, index (col)=0 ("disabled index (col)")) -> (deleted portion=w647:string[][], array with subset deleted=w648:string[][])  [unwired: 1 in]
            n249 = Insert Into Array(array=w648, index (col)=2 ("disabled index (col)"), new element=w647) -> (w638:string[][])  [unwired: 1 in]
            n250 = Build Array(w630, "" ("element"), "" ("element")) -> (w641:string[])
            n251 = Transpose 2D Array(2D array=w638) -> (transposed array=w639:string[][])
            n252 = Insert Into Array(array=w628, new element=w630) -> (w618:string[])  [unwired: 1 in]
            n253 = local read "delimiter"() -> (w635:string)
            n254 = call-poly <vilib>:"Write To Spreadsheet File.vi"("2D data"=dbl[][] [], "file path (dialog if empty)"=w629) -> ("new file path (Not A Path if cancelled)"=w632:path)  [unwired: 6 in]
            n255 = Insert Into Array(array=w639, index (col)=0 ("disabled index (col)"), new element=w641) -> (w634:string[][])  [unwired: 1 in]
            n256 = case shown="True" w613 {
              tunnel: w634 -> [w654 _]
              tunnel: w627 -> [w653 w655]
              tunnel: [w652 w655] -> w622
              frame False {
                n257 = Insert Into Array(array=w653, new element=w654) -> (w652:string[][][])  [unwired: 3 in]
              }
              frame True {
              }
            }
            n258 = Select(t=w626, s=w619, f=w622) -> (s? t:f=w625:string[][][])
            n259 = for {
              tunnel: w632 -> [w660]
              tunnel: w635 -> [w659]
              tunnel: w622 -> [w658] mode=indexing
              tunnel: [FALSE ("Value")] -> w631
              n260 = call-poly <vilib>:"Write To Spreadsheet File.vi"("delimiter (\\t)"=w659, "append to file? (new file:F)"=TRUE, "2D data"=w658, "file path (dialog if empty)"=w660) -> ()  [unwired: 4 in, 1 out]
            }
            n261 = Select(t=w624, s=w619, f=w618) -> (s? t:f=w623:string[])
            n262 = Select(t=w622, s=w619, f=w621) -> (s? t:f=w620:string[][][])
            n263 = property on="Ok" class="Bool (strict)"("Value"=w631) -> ()  [unwired: 2 in, 2 out]
            n264 = Select(t=w618, s=w619, f=w617) -> (s? t:f=w616:string[])
          }
        }
      }
      event "Soglia.ANNULLA": Value Change {
        n265 = event-data() -> ("NewVal"=w672:bool)  [unwired: 1 in]
        n266 = case shown="True" w672 {
          frame False {
          }
          frame True {
            n267 = local read "Grandezze misurate"() -> (w675:i32)
            n268 = property on="Grandezze misurate" class="LstBox (strict)"("Val(Sgnl)"=w675) -> ()  [unwired: 2 in, 2 out]
          }
        }
      }
      event "Soglia interpolata.ANNULLA": Value Change {
        n269 = event-data() -> ("NewVal"=w687:bool)  [unwired: 1 in]
        n270 = case shown="True" w687 {
          frame False {
          }
          frame True {
            n271 = local read "Grandezze misurate"() -> (w690:i32)
            n272 = property on="Grandezze misurate" class="LstBox (strict)"("Val(Sgnl)"=w690) -> ()  [unwired: 2 in, 2 out]
          }
        }
      }
      event "Selezione\nsoglie": Value Change {
        n273 = event-data() -> ("NewVal"=w705:bool)  [unwired: 1 in]
        n274 = call "Vi ref & panel update.vi"("Function"=enum16{"INITIALIZE", "DEF UPDATE"}."DEF UPDATE", "Defer Panel Updates"=TRUE) -> ("error out"=w711:errorcluster)  [unwired: 8 in, 1 out]
        n275 = local read "Grandezze misurate"() -> (w706:i32)
        n276 = property on="Grandezze misurate" class="LstBox (strict)"("Val(Sgnl)"=w706) -> ()  [unwired: 2 in, 2 out]
        n277 = Not(x=w705) -> (.not. x?=w713:bool)
        n278 = property on="Soglia" class="Clust (strict)"(error in=w711, "Visible"=w705) -> (error out=w709:errorcluster)  [unwired: 1 in, 1 out]
        n279 = property on="Soglia interpolata" class="Clust (strict)"(error in=w711, "Visible"=w713) -> (error out=w708:errorcluster)  [unwired: 1 in, 1 out]
        n280 = Merge Errors(w709, w708) -> (w707:errorcluster)
        n281 = call "Vi ref & panel update.vi"("Function"=enum16{"INITIALIZE", "DEF UPDATE"}."DEF UPDATE", "error in (no error)"=w707, "Defer Panel Updates"=FALSE) -> ()  [unwired: 7 in, 2 out]
      }
    }
  }
  n282 = property on="Grandezza riferimento" class="Ring (strict)"("Strings []"=w1) -> ()  [unwired: 2 in, 2 out]
  n283 = invoke class="VI" method="FP.Close"(reference=w17) -> ()  [unwired: 2 in, 3 out]
